vi "LIA Vrms2 to dBm Complex.vi"(11 "Power Spectrum / PSD in":cluster{"f0":dbl, "df":dbl, "magnitude":dbl[]}) -> (3 "Power Spectrum / PSD out":cluster{"f0":dbl, "df":dbl, "magnitude":dbl[]})   [LabVIEW 2018]
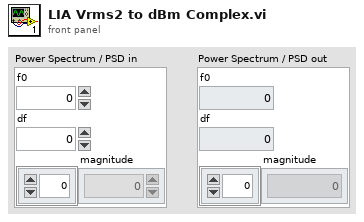
[diagram p1: front panel]
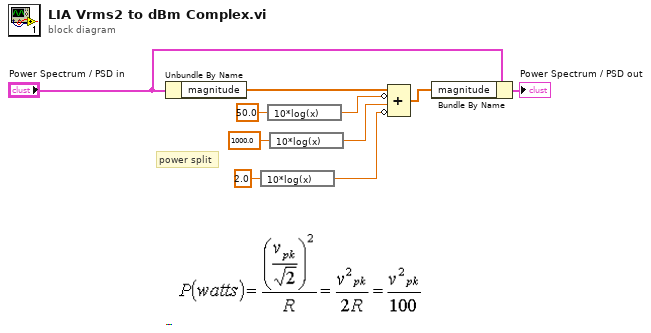
[diagram p0: block diagram]
diagram:
  # "power split"
  n1 = Unbundle By Name("Power Spectrum / PSD in") -> ("magnitude"=w4:dbl[])
  n2 = expression code="10*log(x)"(2.0) -> (w1:dbl)
  n3 = expression code="10*log(x)"(50.0) -> (w7:dbl)
  n4 = expression code="10*log(x)"(1000.0) -> (w10:dbl)
  n5 = Compound Arithmetic op=ADD(w4, invert w7, w10, invert w1) -> (w6:dbl[])
  n6 = Bundle By Name(cluster="Power Spectrum / PSD in", "magnitude"=w6) -> (→"Power Spectrum / PSD out":cluster{"f0":dbl, "df":dbl, "magnitude":dbl[]})
